vi "util_generate_error.vi"(8 "error in (no error)":errorcluster, 9 "show_call_chain":bool=TRUE, 10 "data":variant, 11 "data_error":T1) -> (0 "error out":errorcluster)   [LabVIEW 2015, in "lv-waitgroup.lvlib"]
uses:
  lv-waitgroup.lvlib
  _controls/data_error.ctl
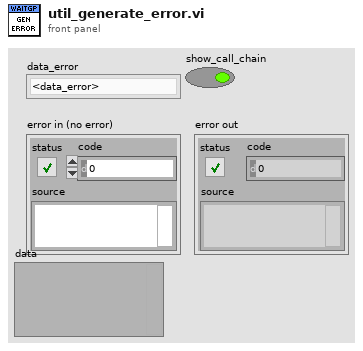
[diagram p1: front panel]
types:
  T1 = typedef "lv-waitgroup.lvlib/data_error.ctl" = enum16{"<data_error>", "unable_to_generate_id", "waitgroup_not_found", "<null>"}
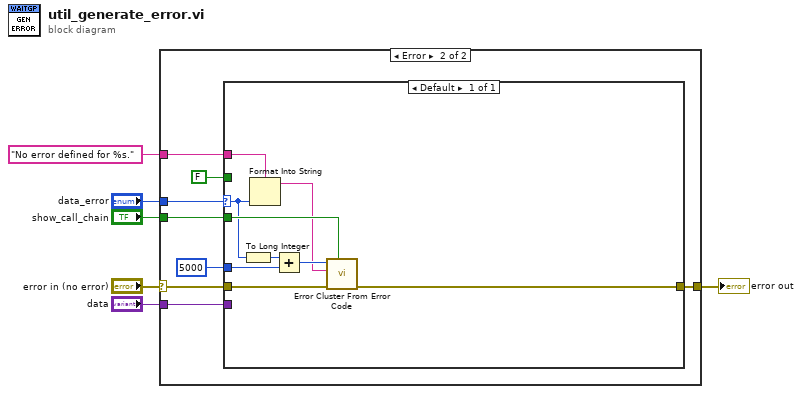
[diagram p0: block diagram]
diagram:
  n1 = case shown="Error" "error in (no error)" {
    selector: "error in (no error)" -> [w7 w15]
    tunnel: [w7 w13] -> w5
    tunnel: "data_error" -> [_ w14]
    tunnel: "show_call_chain" -> [_ w10]
    tunnel: "No error defined for %s." -> [_ w9]
    tunnel: "data" -> [_ w8]
    frame No Error {
    }
    frame Error {
      n2 = case shown="Default" w14 {
        selector: w14 -> [w20]
        tunnel: w15 -> [w24]
        tunnel: [w23] -> w13
        tunnel: 5000 -> [w21]
        tunnel: FALSE -> [_]
        tunnel: w10 -> [w22]
        tunnel: w9 -> [w17]
        tunnel: w8 -> [_]
        frame Default {
          n3 = To Long Integer(number=w20) -> (32bit integer=w19:i32)
          n4 = Format Into String(format string=w17, w20) -> (resulting string=w16:string)  [unwired: 2 in, 1 out]
          n5 = Add(x=w19, y=w21) -> (x+y=w18:i32)
          n6 = call <vilib>:"Error Cluster From Error Code.vi"("show call chain? (False)"=w22, "error in (no error)"=w24, "error message (\"\")"=w16, "error code (0)"=w18) -> ("error out"=w23:errorcluster)  [unwired: 5 in]
        }
      }
    }
  }
  "error out" <- w5
